vi "Timer Main.vi"() -> ()   [LabVIEW 2015]
doc: "This template is for the Queued Message Handler design pattern.\n\nThe Event Handling Loop generates messages based on user interface actions.\n\nThe Message Handling Loop processes messages generated by the Event Handling Loop, or by other messages. The messages are string values, so new messages can be added easily to the Message Cases case structure in the Message Handling Loop. Each message cluster can also provide an optional value for Message Data, which is a variant that can be converted to whatever message-specific data is required."
uses:
  controls/Timer UI Data.ctl
  support/Message Queue/Enqueue Message (Single).vi
  support/Message Queue/Enqueue Message (Array).vi
  <vilib>/Utility/error.llb/Error Cluster From Error Code.vi
  <vilib>/ErrorRing/Error Ring.xnode
  support/Message Queue/Timer Message Queue.lvlib
  support/User Event - Stop/Timer User Event - Stop.lvlib
panel:
  out "Target reached?":bool
  in  "Target Time":dbl=5.23
  out "Elapsed Time":dbl
  in  "Stop 2":bool
  out "Display":string
  in  "Reset":bool
  in  "Start":bool
  in  "Exit":bool
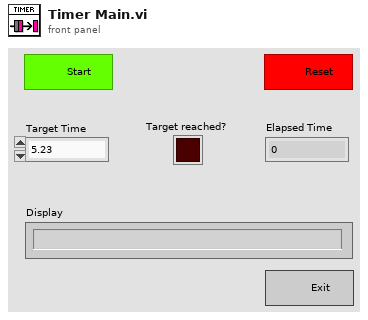
[diagram p1: front panel]
types:
  T1 = typedef "Timer UI Data.ctl" = cluster{"Boolean <Replace Me>":bool, "String <Replace Me>":string, "Numeric <Replace Me>":dbl, "Do Something Ref":refnum<vi>, "Do Something Else Ref":refnum<vi>, "Data Display Ref":refnum<vi>, "Exit Button Ref":refnum<vi>}
  T2 = typedef "Timer Message Queue.lvlib/All Message Queues.ctl" = cluster{"UI":refnum<queue>}
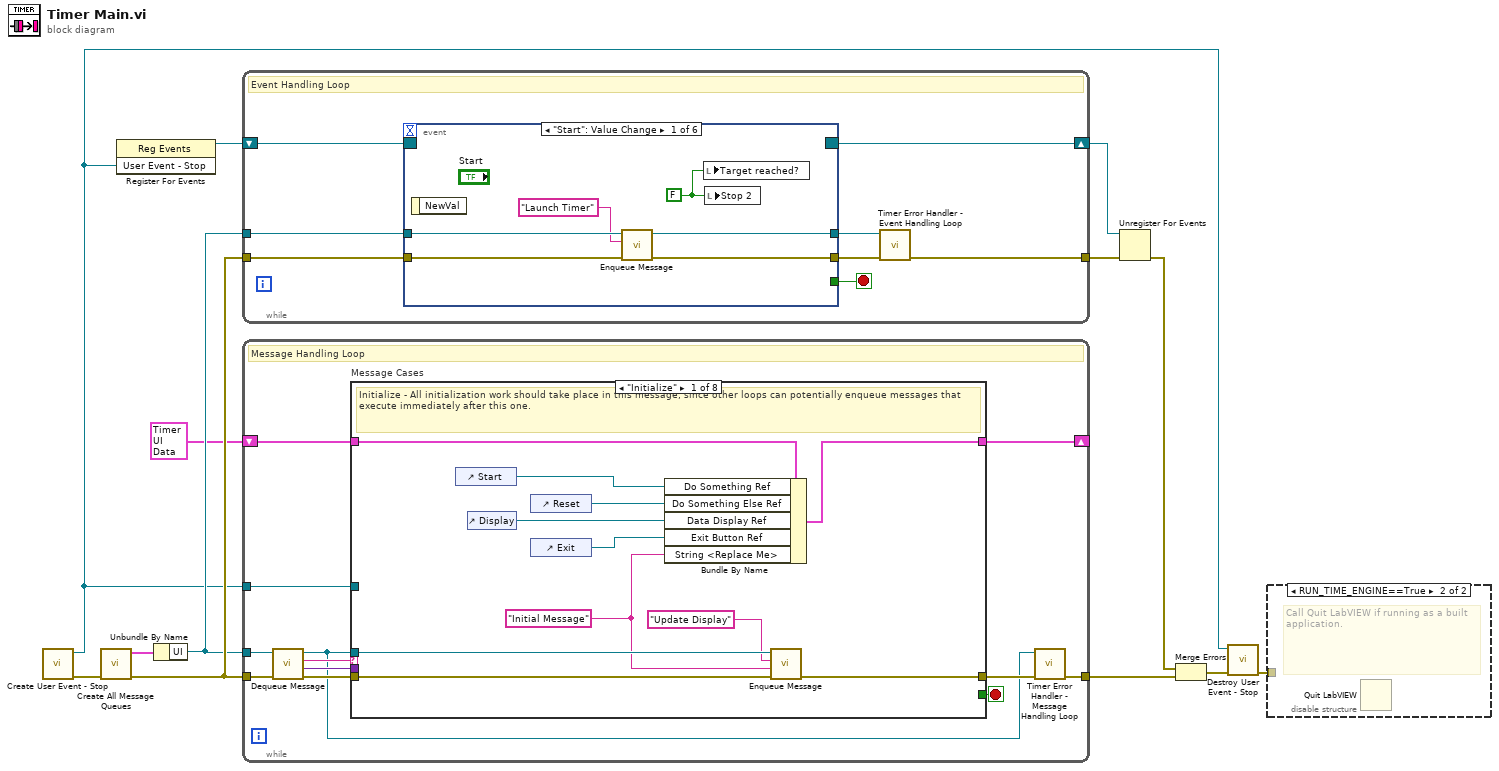
[diagram p0: block diagram]
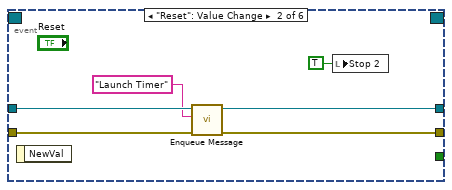
[diagram p3: hidden frame]
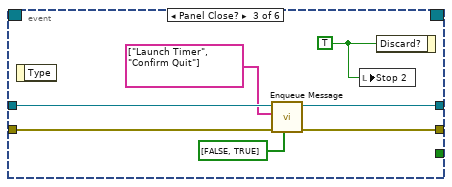
[diagram p4: hidden frame]
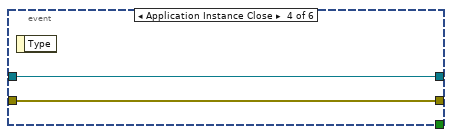
[diagram p5: hidden frame]
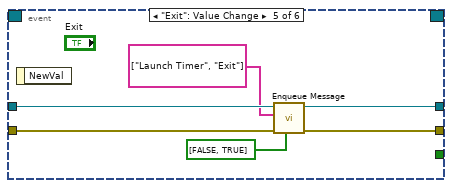
[diagram p6: hidden frame]
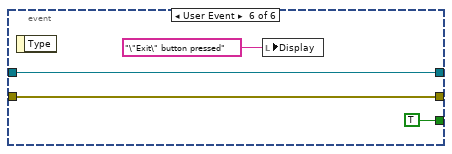
[diagram p7: hidden frame]
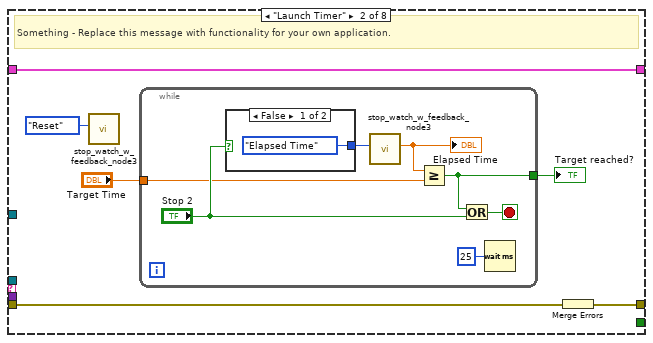
[diagram p8: hidden frame]
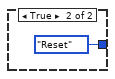
[diagram p9: hidden frame]
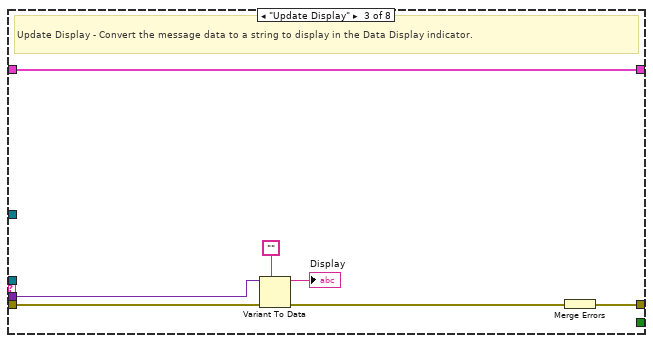
[diagram p10: hidden frame]
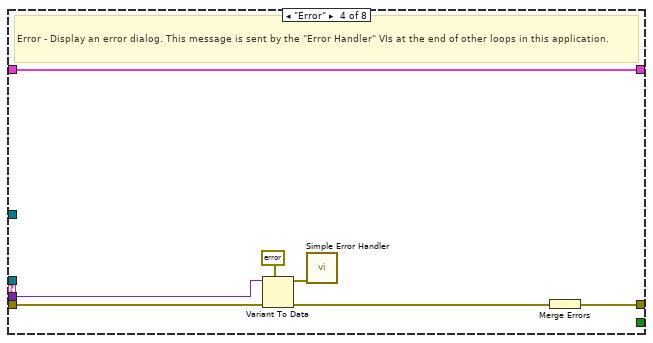
[diagram p11: hidden frame]
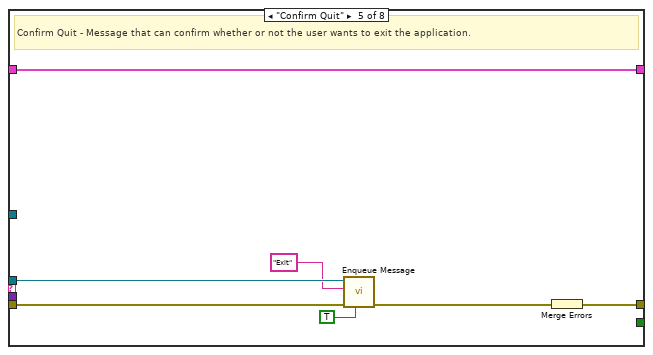
[diagram p12: hidden frame]
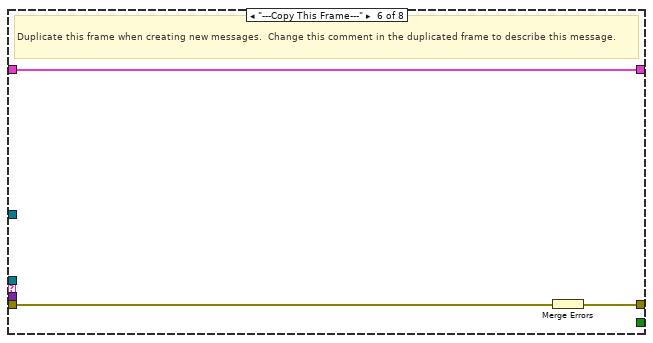
[diagram p13: hidden frame]
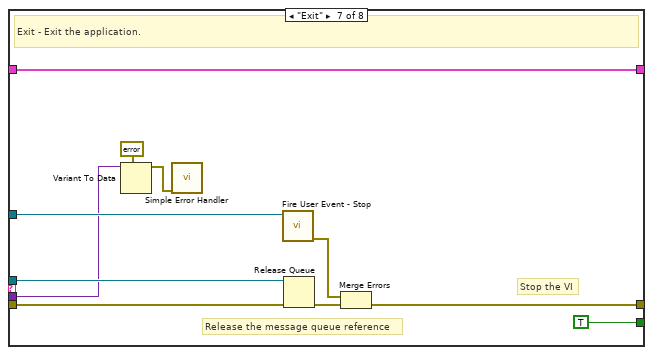
[diagram p14: hidden frame]
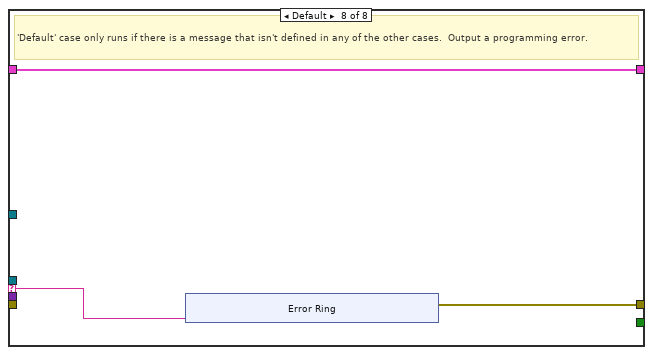
[diagram p15: hidden frame]
diagram:
  n1 = call "Create User Event - Stop.vi"() -> ("error out"=w9:errorcluster, "User Event - Stop"=w1:refnum<user-event>)  [unwired: 10 in]
  n2 = call "Create All Message Queues.vi"("error in (no error)"=w9) -> ("error out"=w13:errorcluster, "Message Queues out"=w12:T2)  [unwired: 9 in]
  n3 = register-events(w1) -> (reference out=w3:refnum<event-registration>)  [unwired: 2 in, 1 out]
  n4 = Unbundle By Name(w12) -> ("UI"=w10:refnum<queue>)
  n5 = while {
    tunnel: w10 -> [w21]
    shift-right: [w19] -> w7
    shift-left: w3 -> [w20]
    tunnel: [w15] -> w4
    tunnel: w13 -> [w14]
    stop <- w17 stop-if-true
    # "Event Handling Loop"
    n6 = event shown="[0] \"Start\": Value Change" {
      selector: w20 -> [_ _ _ _ _ _]
      dyn-events: [_ _ _ _ _ _] -> w19
      timeout: _ -> [_ _ _ _ _ _]
      tunnel: [_ _ _ _ _ TRUE ("Discard?")] -> w17
      tunnel: w21 -> [w27 w33 w40 w42 w48 w52]
      tunnel: [w24 w30 w39 w41 w47 w49] -> w18
      tunnel: [w26 w32 w38 w42 w46 w52] -> w16
      tunnel: w14 -> [w23 w29 w37 w41 w45 w49]
      event "Start": Value Change {
        w22 = FALSE ("Stop 2")
        n7 = event-data() -> ()  [unwired: 1 in, 1 out]
        n8 = call-poly "Enqueue Message.vi"("error in (no error)"=w23, "Message"="Launch Timer", "Message Queue"=w27) -> ("error out"=w24:errorcluster, "dup Message Queue"=w26:refnum<queue>)  [unwired: 7 in]
        n9 = local write "Target reached?"(w22) -> ()
        n10 = local write "Stop 2"(w22) -> ()
      }
      event "Reset": Value Change {
        n11 = event-data() -> ()  [unwired: 1 in, 1 out]
        n12 = call-poly "Enqueue Message.vi"("error in (no error)"=w29, "Message"="Launch Timer", "Message Queue"=w33) -> ("error out"=w30:errorcluster, "dup Message Queue"=w32:refnum<queue>)  [unwired: 7 in]
        n13 = local write "Stop 2"(TRUE ("Stop 2")) -> ()
      }
      event Panel Close? {
        w34 = TRUE ("Discard?")
        n14 = event-data() -> ()  [unwired: 1 in, 1 out]
        n15 = call-poly "Enqueue Message.vi"("Priority Message? Array"=bool[] [FALSE, TRUE], "error in (no error)"=w37, "Message Array"=string[] ["Launch Timer", "Confirm Quit"], "Message Queue"=w40) -> ("error out"=w39:errorcluster, "dup Message Queue"=w38:refnum<queue>)  [unwired: 6 in]
        n16 = local write "Stop 2"(w34) -> ()
        n17 = event-data("Discard?"=w34) -> ()  [unwired: 1 in, 1 out]
      }
      event Application Instance Close {
        n18 = event-data() -> ()  [unwired: 1 in, 1 out]
      }
      event "Exit": Value Change {
        n19 = event-data() -> ()  [unwired: 1 in, 1 out]
        n20 = call-poly "Enqueue Message.vi"("Priority Message? Array"=bool[] [FALSE, TRUE], "error in (no error)"=w45, "Message Array"=string[] ["Launch Timer", "Exit"], "Message Queue"=w48) -> ("error out"=w47:errorcluster, "dup Message Queue"=w46:refnum<queue>)  [unwired: 6 in]
      }
      event User Event {
        n21 = event-data() -> ()  [unwired: 1 in, 1 out]
        n22 = local write "Display"("\"Exit\" button pressed" ("VI Stopped")) -> ()
      }
    }
    n23 = call "Timer Error Handler - Event Handling Loop.vi"("error in (no error)"=w18, "Message Queue"=w16) -> ("dup error in"=w15:errorcluster)  [unwired: 8 in, 1 out]
  }
  n24 = while {
    tunnel: w10 -> [w56]
    shift-right: [w63] -> _
    shift-left: T1 {"Boolean <Replace Me>"=FALSE, "String <Replace Me>"="", "Numeric <Replace Me>"=0.0, "Do Something Ref"=refnum, "Do Something Else Ref"=refnum, "Data Display Ref"=refnum, "Exit Button Ref"=refnum} ("Data Cluster") -> [w64]
    tunnel: w1 -> [w61]
    tunnel: w13 -> [w60]
    tunnel: [w55] -> w11
    stop <- w62 stop-if-true
    # "Message Handling Loop"
    n25 = call "Dequeue Message.vi"("error in (no error)"=w60, "Message Queue"=w56) -> ("error out"=w59:errorcluster, "Message Data"=w57:variant, "Message"=w58:string, "dup Message Queue"=w53:refnum<queue>)  [unwired: 6 in]
    n26 = case "Message Cases" shown="\"Initialize\"" w58 {
      selector: w58 -> [_ _ _ _ _ _ _ w126]
      tunnel: w53 -> [w67 _ _ _ w107 _ w125 _]
      tunnel: w59 -> [w74 w79 w95 w104 w111 w114 w118 _]
      tunnel: [w75 w80 w96 w98 w109 w112 w121 w127] -> w54
      tunnel: w64 -> [w73 w81 w97 w103 w110 w113 w124 w128]
      tunnel: [w72 w81 w97 w103 w110 w113 w124 w128] -> w63
      tunnel: [_ _ _ _ _ _ TRUE _] -> w62
      tunnel: w57 -> [_ _ w94 w102 _ _ w115 _]
      tunnel: w61 -> [_ _ _ _ _ _ w120 _]
      frame "Initialize" {
        w66 = "Initial Message" ("Initial Message")
        # "Initialize - All initialization work should take place in this message, since other loops can potentially enqueue messages that execute immediately after this one."
        n27 = control-ref of="Start"() -> (w71:refnum<vi>)
        n28 = control-ref of="Display"() -> (w69:refnum<vi>)
        n29 = control-ref of="Reset"() -> (w70:refnum<vi>)
        n30 = control-ref of="Exit"() -> (w68:refnum<vi>)
        n31 = Bundle By Name(cluster=w73, "Do Something Ref"=w71, "Do Something Else Ref"=w70, "Data Display Ref"=w69, "Exit Button Ref"=w68, "String <Replace Me>"=w66) -> (w72:T1)
        n32 = call-poly "Enqueue Message.vi"("error in (no error)"=w74, "Message Data"=w66, "Message"="Update Display", "Message Queue"=w67) -> ("error out"=w75:errorcluster)  [unwired: 6 in, 1 out]
      }
      frame "Launch Timer" {
        # "Something - Replace this message with functionality for your own application."
        n33 = call "stop_watch_w_feedback_node3.vi"("Command"=enum16{"Elapsed Time", "Reset"}."Reset") -> ()  [unwired: 10 in, 1 out]
        n34 = while {
          tunnel: "Target Time" -> [w84]
          tunnel: [w85] -> w76
          stop <- w87 stop-if-true
          n35 = case shown="False" "Stop 2" {
            tunnel: [enum16{"Elapsed Time", "Reset"}."Elapsed Time" ("Command") enum16{"Elapsed Time", "Reset"}."Reset" ("Command")] -> w88
            frame False {
            }
            frame True {
            }
          }
          n36 = call "stop_watch_w_feedback_node3.vi"("Command"=w88) -> ("Elapsed Time"=w83:dbl)  [unwired: 10 in]
          "Elapsed Time" <- w83
          n37 = Greater Or Equal?(x=w83, y=w84) -> (x >= y?=w85:bool)
          n38 = Or(x=w85, y="Stop 2") -> (x .or. y?=w87:bool)
          n39 = Wait (ms)(milliseconds to wait=u32 25) -> ()  [unwired: 1 out]
        }
        "Target reached?" <- w76
        n40 = Merge Errors(w79) -> (w80:errorcluster)
      }
      frame "Update Display" {
        # "Update Display - Convert the message data to a string to display in the Data Display indicator."
        n41 = Variant To Data(error in=w95, type="", Variant=w94) -> (data=→"Display":string, error out=w92:errorcluster)
        n42 = Merge Errors(w92) -> (w96:errorcluster)
      }
      frame "Error" {
        # "Error - Display an error dialog. This message is sent by the \"Error Handler\" VIs at the end of other loops in this application."
        n43 = Variant To Data(error in=w104, type=errorcluster {"status"=FALSE, "code"=0, "source"=""} ("error constant"), Variant=w102) -> (data=w100:errorcluster, error out=w99:errorcluster)
        n44 = call <vilib>:"Simple Error Handler.vi"("error in (no error)"=w100) -> ()  [unwired: 4 in, 5 out]
        n45 = Merge Errors(w99) -> (w98:errorcluster)
      }
      frame "Confirm Quit" {
        # "Confirm Quit - Message that can confirm whether or not the user wants to exit the application."
        n46 = call-poly "Enqueue Message.vi"("Priority Message? (F)"=TRUE, "error in (no error)"=w111, "Message"="Exit", "Message Queue"=w107) -> ("error out"=w108:errorcluster)  [unwired: 6 in, 1 out]
        n47 = Merge Errors(w108) -> (w109:errorcluster)
      }
      frame "---Copy This Frame---" {
        # "Duplicate this frame when creating new messages.  Change this comment in the duplicated frame to describe this message."
        n48 = Merge Errors(w114) -> (w112:errorcluster)
      }
      frame "Exit" {
        # "Stop the VI"
        # "Release the message queue reference"
        # "Exit - Exit the application."
        n49 = Variant To Data(type=errorcluster {"status"=FALSE, "code"=0, "source"=""} ("error constant"), Variant=w115) -> (data=w116:errorcluster)  [unwired: 1 in, 1 out]
        n50 = call <vilib>:"Simple Error Handler.vi"("error in (no error)"=w116) -> ()  [unwired: 4 in, 5 out]
        n51 = call "Fire User Event - Stop.vi"("User Event - Stop"=w120) -> ("error out"=w119:errorcluster)  [unwired: 10 in]
        n52 = Release Queue(queue=w125, error in (no error)=w118) -> (error out=w122:errorcluster)  [unwired: 1 in, 2 out]
        n53 = Merge Errors(w119, w122) -> (w121:errorcluster)
      }
      frame Default {
        # "'Default' case only runs if there is a message that isn't defined in any of the other cases.  Output a programming error."
        n54 = xnode "Error Ring"("parameter 0"=w126) -> ("error out"=w127:errorcluster)
      }
    }
    n55 = call "Timer Error Handler - Message Handling Loop.vi"("error in (no error)"=w54, "Message Queue"=w53) -> ("dup error in"=w55:errorcluster)  [unwired: 8 in, 1 out]
  }
  n56 = Unregister For Events(event registration refnum=w7, error in=w4) -> (error out=w2:errorcluster)
  n57 = Merge Errors(w2, w11) -> (w8:errorcluster)
  n58 = call "Destroy User Event - Stop.vi"("error in (no error)"=w8, "User Event - Stop"=w1) -> ("error out"=w5:errorcluster)  [unwired: 9 in]
  n59 = disable-structure shown="RUN_TIME_ENGINE==True" {
    disable-tunnel: w5 -> [_ _]
    frame condition #0 (active) {
    }
    frame condition #1 {
      # "Call Quit LabVIEW if running as a built application."
      n60 = Quit LabVIEW() -> ()  [unwired: 1 in]
    }
  }
